vi "Patch.vi"(8 "Error In":errorcluster) -> (0 "Error Out":errorcluster)   [LabVIEW 2017, in "Tests.lvlib" / "Version.lvlib"]
uses:
  Version.lvlib
  <vilib>/addons/_JKI Toolkits/Caraya/classes/Test/Test.lvclass
  <vilib>/addons/_JKI Toolkits/Caraya/classes/Assert/Assert.lvclass
  src/LabPack/LabPack.lvlib
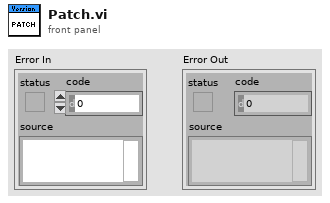
[diagram p1: front panel]
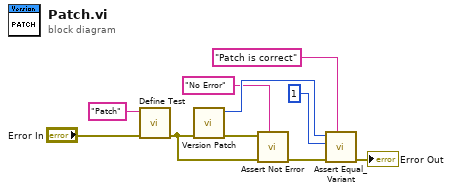
[diagram p0: block diagram]
diagram:
  n1 = call <vilib>:"Define Test.vi"("error in (no error)"="Error In", "Label (VI Title)"="Patch") -> ("error out"=w8:errorcluster)  [unwired: 9 in]
  n2 = call "Version Patch.vi"("Error In"=w8) -> ("Error Out"=w6:errorcluster, "Version Patch"=w4:u32)  [unwired: 9 in]
  n3 = call <vilib>:"Assert Not Error.vi"("Label"="No Error", "error in (no error)"=w8, "Not Error?"=w6) -> ("error out"=w7:errorcluster)  [unwired: 8 in]
  n4 = call <vilib>:"Assert Equal_Variant.vi"("Label"="Patch is correct", "error in (no error)"=w7, "Y"=u32 1 ("Version Major"), "X"=w4) -> ("error out"=→"Error Out":errorcluster)  [unwired: 7 in]
